vi "Get Property.vi"(0 "Properties":map{string, string}(c390), 5 "Property Name":string, 11 "error in":errorcluster) -> (4 "Non-empty Value Found":bool, 6 "Value":string, 15 "error out":errorcluster)   [LabVIEW 2023]
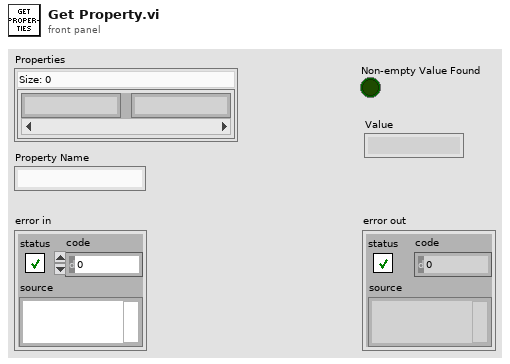
[diagram p1: front panel]
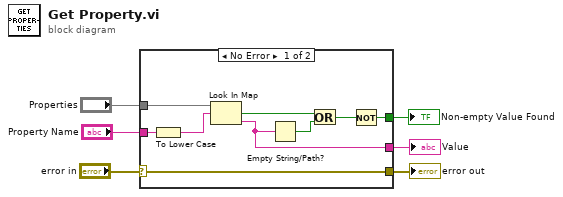
[diagram p0: block diagram]
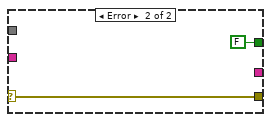
[diagram p2: hidden frame]
diagram:
  n1 = case shown="No Error" "error in" {
    selector: "error in" -> [w8 w17]
    tunnel: "Property Name" -> [w15 _]
    tunnel: "Properties" -> [w11 _]
    tunnel: [w9 FALSE] -> w4
    tunnel: [w8 w17] -> w2
    tunnel: [w7 _] -> w1
    frame No Error {
      n2 = To Lower Case(string=w15) -> (all lower case string=w12:string)
      n3 = Look In Map(map=w11, key=w12) -> (key not found?=w14:bool, value=w7:string)  [unwired: 1 in]
      n4 = Empty String/Path?(string/path=w7) -> (empty?=w13:bool)
      n5 = Or(x=w14, y=w13) -> (x .or. y?=w10:bool)
      n6 = Not(x=w10) -> (.not. x?=w9:bool)
    }
    frame Error {
    }
  }
  "Non-empty Value Found" <- w4
  "error out" <- w2
  "Value" <- w1
